vi "drive_turn.vi"(5 "reset":bool, 7 "turn_hdg":dbl, 8 "gyro_angle":dbl, 10 "speed_right":dbl) -> (1 "done":bool, 2 "right":dbl, 3 "left":dbl)   [LabVIEW 2014]
panel:
  in  "finish_timer":u8
  in  "finish_thresh":dbl
  in  "angle_ki":dbl
  in  "angle_kp":dbl
  out "pi_settle_timer":u8(graph)
  out "pi_output":dbl(graph)
  out "pi_integral":dbl(graph)
  out "angle":dbl(graph)
  in  "lock_ki":dbl
  in  "lock_kp":dbl
  out "pi_output":dbl(graph)
  out "pi_integral":dbl(graph)
  out "spd_error":dbl(graph)
  # "Inner Wheel Lock - PI Speed Control"
  # "Outer Wheel Angular Control - PI angular control"
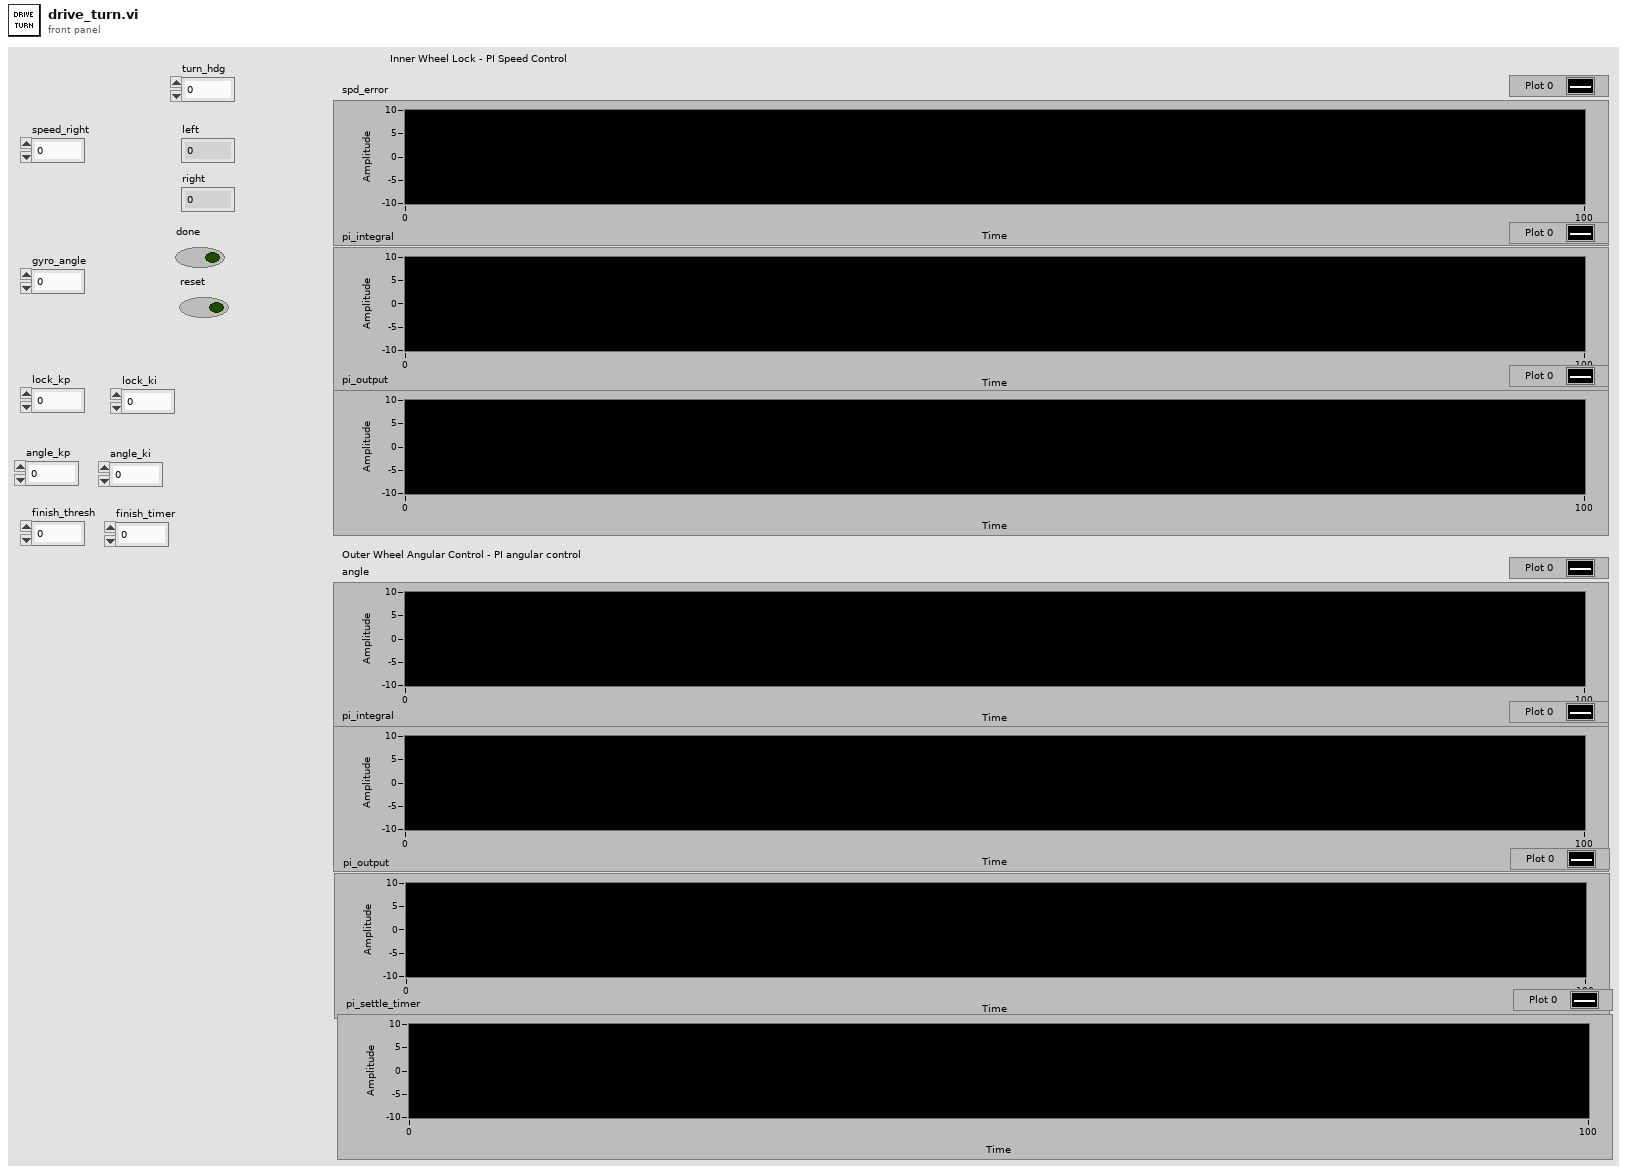
[diagram p1: front panel]
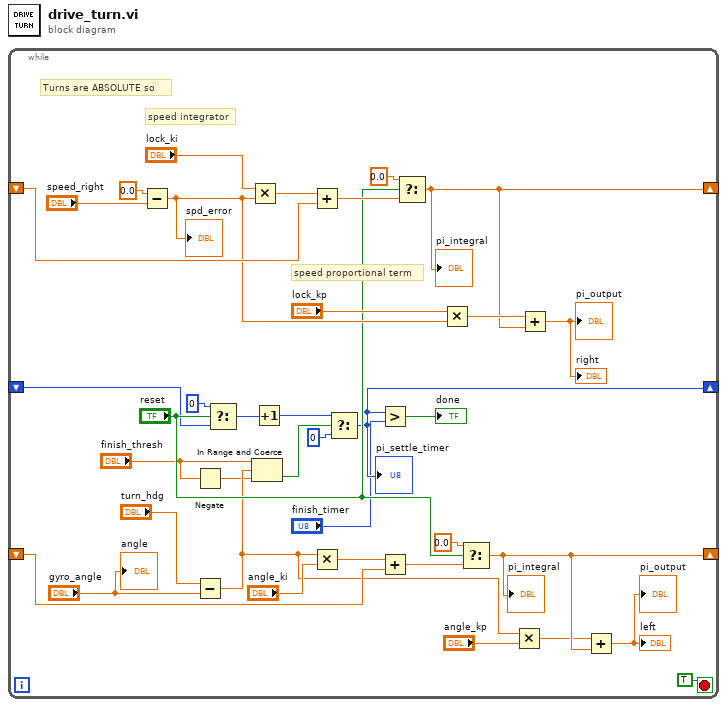
[diagram p0: block diagram]
diagram:
  n1 = while {
    shift-right: [w27] -> _
    shift-left: _ -> [w32]
    shift-right: [w17] -> _
    shift-left: _ -> [w20]
    shift-right: [w4] -> _
    shift-left: _ -> [w12]
    stop <- TRUE stop-if-true
    # "Turns are ABSOLUTE so"
    # "speed integrator"
    # "speed proportional term"
    n2 = Subtract(x=0.0, y="speed_right") -> (x-y=w28:dbl)
    "spd_error" <- w28
    n3 = Negate(x="finish_thresh") -> (-x=w10:dbl)
    n4 = Subtract(x="turn_hdg", y="gyro_angle") -> (x-y=w11:dbl)
    n5 = Select(t=u8 0, s="reset", f=w12) -> (s? t:f=w6:u8)
    n6 = Multiply(x="lock_ki", y=w28) -> (x*y=w33:dbl)
    n7 = In Range and Coerce(upper limit="finish_thresh", x=w11, lower limit=w10) -> (In Range?=w8:bool)  [unwired: 1 out]
    n8 = Increment(x=w6) -> (x+1=w7:u8)
    n9 = Add(x=w33, y=w32) -> (x+y=w31:dbl)
    n10 = Multiply(x=w11, y="angle_ki") -> (x*y=w18:dbl)
    n11 = Select(t=w7, s=w8, f=u8 0) -> (s? t:f=w4:u8)
    "pi_settle_timer" <- w4
    n12 = Greater?(x=w4, y="finish_timer") -> (0:→"done":bool)
    n13 = Add(x=w18, y=w20) -> (x+y=w21:dbl)
    n14 = Select(t=0.0, s="reset", f=w31) -> (s? t:f=w27:dbl)
    "pi_integral" <- w27
    n15 = Multiply(x="lock_kp", y=w28) -> (x*y=w29:dbl)
    n16 = Select(t=0.0, s="reset", f=w21) -> (s? t:f=w17:dbl)
    "pi_integral" <- w17
    n17 = Multiply(x=w11, y="angle_kp") -> (x*y=w16:dbl)
    n18 = Add(x=w29, y=w27) -> (x+y=→"right" →"pi_output":dbl)
    n19 = Add(x=w16, y=w17) -> (x+y=→"left" →"pi_output":dbl)
    "angle" <- "gyro_angle"
  }
